vi "Cryocon Get Data.vi"(2 "Point #":i32, 3 "Command String":string, 4 "GPIB Address":refnum<visa-resource-name>) -> (0 "Stop":bool, 1 "Measurement":dbl[](array[numeric]) format="%.2e")   [LabVIEW 2024]
doc: "This VI reads a single reading from a Keithley 2001 multimeter. The stop boolean is always false. If no reading is obtained a single zero is returned.\nScott Hannahs, NHMFL-FSU, Nov 1993"
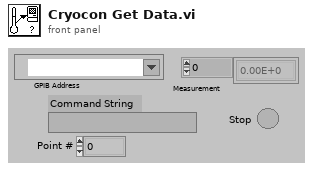
[diagram p1: front panel]
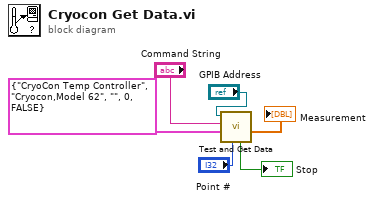
[diagram p0: block diagram]
diagram:
  n1 = call "Test and Get Data.vi"("Point #"="Point #", "Instrument Info"=cluster{string, string, string, u32, bool} {"CryoCon Temp Controller", "Cryocon,Model 62", "", 0, FALSE}, "Command String"="Command String", "VISA Sesson"="GPIB Address") -> ("Measurement"=→"Measurement":dbl[], "Stop"=→"Stop":bool)  [unwired: 2 in, 3 out]
